vi "putFile.vi"(8 "error in (no error)":errorcluster, 9 "local path":path, 10 "remote path":string, 11 "ConnectionData":T1) -> (0 "error out":errorcluster, 3 "local path out":path)   [LabVIEW 2015]
uses:
  connectionData.ctl
panel:
  # "Puts a file to a remote location. Uses the pscp utility to perform the\ntransfer. This VI expects to find pscp.exe in the same dirctory that\nthis VI is located in.\nDOWNLOAD: http://www.chiark.greenend.org.uk/~sgtatham/putty/download.html"
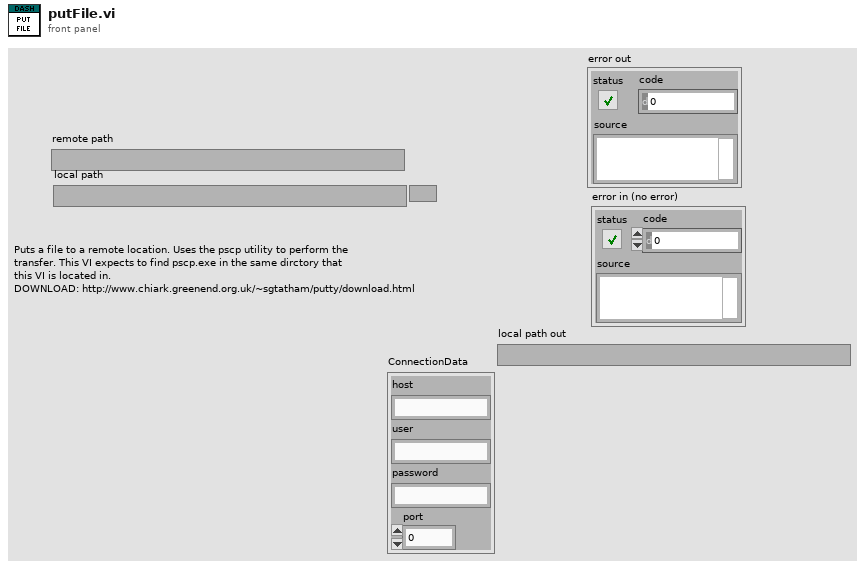
[diagram p1: front panel]
types:
  T1 = typedef "connectionData.ctl" = cluster{"host":string, "user":string, "password":string, "port":u16}
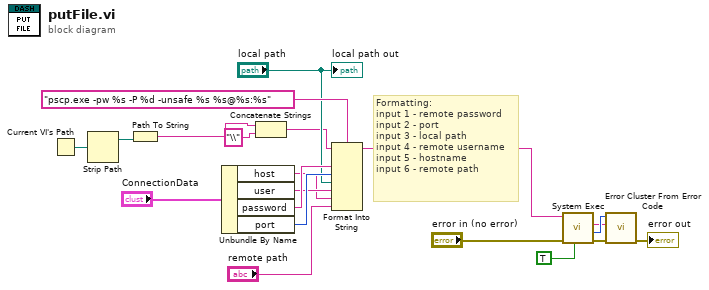
[diagram p0: block diagram]
diagram:
  # "Formatting:\ninput 1 - remote password\ninput 2 - port\ninput 3 - local path\ninput 4 - remote username\ninput 5 - hostname\ninput 6 - remote path"
  n1 = Current VI's Path() -> (path=w18:path)
  n2 = Strip Path(path=w18) -> (stripped path=w2:path)  [unwired: 1 out]
  n3 = Path To String(path=w2) -> (string=w1:string)
  n4 = Unbundle By Name("ConnectionData") -> ("host"=w7:string, "user"=w8:string, "password"=w11:string, "port"=w10:u16)
  n5 = Concatenate Strings(w1, "\\" ("string")) -> (w3:string)
  n6 = Format Into String(format string="pscp.exe -pw %s -P %d -unsafe %s %s@%s:%s", initial string=w3, w11, w10, "local path", w8, w7, "remote path") -> (resulting string=w5:string)  [unwired: 1 in, 1 out]
  n7 = call <vilib>:"System Exec.vi"("run minimized? (F)"=TRUE, "error in (no error)"="error in (no error)", "command line"=w5) -> ("error out"=w13:errorcluster, "return code"=w17:i32, "standard error"=w16:string)  [unwired: 5 in, 1 out]
  n8 = call <vilib>:"Error Cluster From Error Code.vi"("error in (no error)"=w13, "error message (\"\")"=w16, "error code (0)"=w17) -> ("error out"=→"error out":errorcluster)  [unwired: 6 in]
  "local path out" <- "local path"
